vi "Create.vi"(3 "Parent Name":string) -> (1 "Redlines Identity out":refnum<class "Redlines Identity.lvclass">)   [LabVIEW 2020, in "VolatusData.lvlib" / "Redlines Identity.lvclass"]
uses:
  Redlines Identity.lvclass
  Redlines Identity.lvclass/Redlines Identity.ctl
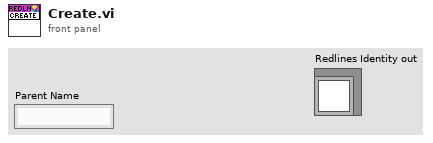
[diagram p1: front panel]
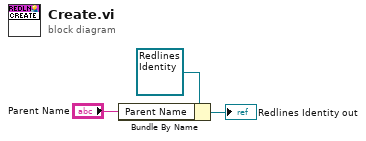
[diagram p0: block diagram]
diagram:
  n1 = Bundle By Name(cluster=refnum<class "Redlines Identity.lvclass"> refnum ("DataProc Identity in"), "Parent Name"="Parent Name") -> (→"Redlines Identity out":refnum<class "Redlines Identity.lvclass">)
